vi "Get Data.vi"() -> (3 "Data Out":i32[](array[numeric]))   [LabVIEW 2019, in "Custom Calendar.xctl"]
uses:
  Custom Calendar.xctl
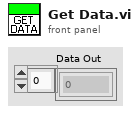
[diagram p1: front panel]
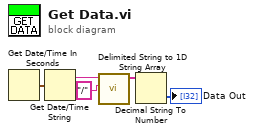
[diagram p0: block diagram]
diagram:
  n1 = Get Date/Time In Seconds() -> (seconds since 1Jan1904=w5:timestamp)
  n2 = Get Date/Time String(seconds (now)=w5) -> (date string=w4:string)  [unwired: 2 in, 1 out]
  n3 = call <vilib>:"Delimited String to 1D String Array.vi"("delimiter"="/", "delimited string"=w4) -> ("string array"=w2:string[])  [unwired: 9 in]
  n4 = Decimal String To Number(string=w2) -> (number=→"Data Out":i32[])  [unwired: 2 in, 1 out]
